vi "Read Type.vi"(8 "Error In":errorcluster, 11 "Datum In":refnum<class "Datum.lvclass">) -> (0 "Error Out":errorcluster, 2 "Type":T1=enum."Unknown", 3 "Datum Out":refnum<class "Datum.lvclass">)   [LabVIEW 2018, in "Toolkit.lvlib" / "Data.lvlib" / "Datum.lvclass"]
doc: "Gets the Mustache data type of an object. This is primarily used internally or when building custom compilers. This is more robust than using strings in case structures with the Get LV Class Name function, which is not available in older versions of LabVIEW.\n\n<B>Datum In/Out</B> - Represents a Mustache data value.\n\n<B>Type</B> - Indicates the data type as an enum. This is useful when the Get LV Class Name function is not available."
uses:
  Datum.lvclass
  Type Defintions/Types.ctl
  Data.lvlib
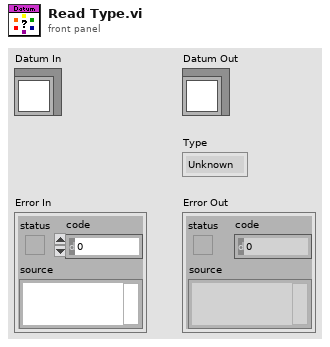
[diagram p1: front panel]
types:
  T1 = typedef "Toolkit.lvlib/Data.lvlib/Types.ctl" = enum16{"Array", "Boolean", "Function", "Map", "Null", "Pair", "Path", "String", "Unknown"}
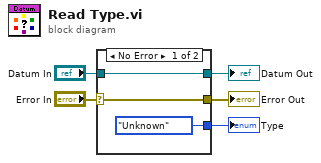
[diagram p0: block diagram]
diagram:
  n1 = case shown="No Error" "Error In" {
    selector: "Error In" -> [w7 w10]
    tunnel: [w7 w10] -> w4
    tunnel: [w8 w9] -> w2
    tunnel: "Datum In" -> [w8 w9]
    tunnel: [Types."Unknown" ("Type") _] -> w1
    frame No Error {
    }
    frame Error {
    }
  }
  "Error Out" <- w4
  "Datum Out" <- w2
  "Type" <- w1
